vi "Add Multiple Items to End.vi"(8 "error in (no error)":errorcluster, 10 "Items":T1(array[cluster]), 11 "FastTreeView in":refnum<class "FastTreeView.lvclass">) -> (0 "error out":errorcluster, 3 "FastTreeView out":refnum<class "FastTreeView.lvclass">)   [LabVIEW 2025, in "FastTreeView.lvclass"]
uses:
  FastTreeView.lvclass
  FastTreeView.lvclass/FastTreeView.ctl
  C:/Git/FastTreeView/FastTreeView/LV/FastTreeView/dll/FastTreeView.dll
  dll/FastTreeView.dll
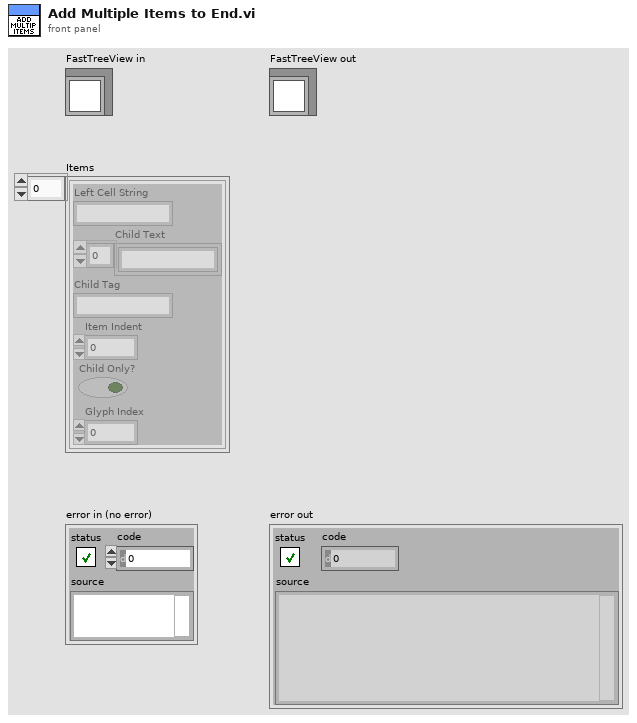
[diagram p1: front panel]
types:
  T1 = cluster{"Left Cell String":string, "Child Text":string[], "Child Tag":string, "Item Indent":i32, "Child Only?":bool, "Glyph Index":i32}[]
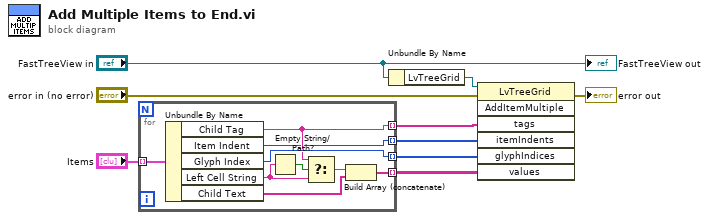
[diagram p0: block diagram]
diagram:
  n1 = for {
    tunnel: "Items" -> [w18] mode=indexing
    tunnel: [w11] -> w4 mode=indexing
    tunnel: [w16] -> w3 mode=indexing
    tunnel: [w15] -> w2 mode=indexing
    tunnel: [w10] -> w1 mode=indexing
    n2 = Unbundle By Name(w18) -> ("Child Tag"=w11:string, "Item Indent"=w10:i32, "Glyph Index"=w15:i32, "Left Cell String"=w13:string, "Child Text"=w17:string[])
    n3 = Empty String/Path?(string/path=w13) -> (empty?=w14:bool)
    n4 = Select(t=w11, s=w14, f=w13) -> (s? t:f=w12:string)
    n5 = Build Array (concatenate)(w12, w17) -> (w16:string[])
  }
  n6 = Unbundle By Name("FastTreeView in") -> ("LvTreeGrid"=w8:refnum<k24>)
  n7 = invoke class="LvTreeGrid" method="AddItemMultiple"(reference=w8, error in="error in (no error)", "tags"=w4, "itemIndents"=w1, "glyphIndices"=w2, "values"=w3) -> (error out=→"error out":errorcluster)  [unwired: 1 in, 6 out]
  "FastTreeView out" <- "FastTreeView in"
